vi "Begin.vi"() -> (0 "error out":errorcluster)   [LabVIEW 2013]
doc: "Called before other user functions, this VI is expected to open initial I/O refnums, load in file data, and do all program initialization. Notice that the <B>error out</B> terminal is simply used for data flow. Wiring it to other structures or subVIs ensures that this VI runs first."
uses:
  <vilib>/Rock Robotics/SystemInterfaces/DIO/FPGA_DIOPWMChannel.ctl
  <vilib>/Rock Robotics/WPI/DriverStation/WPI_DriverStationRobotMode2.ctl
  <vilib>/Rock Robotics/WPI/Joystick/WPI_JoystickDeviceEnum.ctl
  <vilib>/Rock Robotics/WPI/SafetyOutput/WPI_SafetyOutputConfigMenu.ctl
  <vilib>/Rock Robotics/SystemInterfaces/DIO/FPGA_DIORelayChannel.ctl
  <vilib>/Rock Robotics/SystemInterfaces/DIO/FPGA_DIOChannel.ctl
  <vilib>/Rock Robotics/SystemInterfaces/Typedef/FPGA_TypedefDigitalModule.ctl
  <vilib>/Rock Robotics/WPI/RobotDrive/WPI_RobotDriveOpen2MotorWithTalon.vi
  Robot Global Data.vi
  <vilib>/Rock Robotics/WPI/Compressor/WPI_CompressorGetSetRefNum.vi
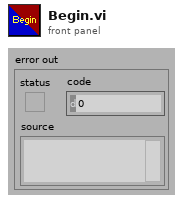
[diagram p1: front panel]
types:
  T1 = typedef "FPGA_TypedefDigitalModule.ctl" = enum16{"Digital Module 1", "Digital Module 2"}
  T2 = typedef "FPGA_DIOChannel.ctl" = enum8{"DIO 1", "DIO 2", "DIO 3", "DIO 4", "DIO 5", "DIO 6", "DIO 7", "DIO 8", "DIO 9", "DIO 10", "DIO 11", "DIO 12", "DIO 13", "DIO 14", "Invalid"}
  T3 = typedef "FPGA_DIORelayChannel.ctl" = enum8{"Relay 1", "Relay 2", "Relay 3", "Relay 4", "Relay 5", "Relay 6", "Relay 7", "Relay 8", "Invalid"}
  T4 = typedef "WPI_SafetyOutputConfigMenu.ctl" = enum16{"Enable", "Disable"}
  T5 = typedef "FPGA_DIOPWMChannel.ctl" = enum8{"PWM 1", "PWM 2", "PWM 3", "PWM 4", "PWM 5", "PWM 6", "PWM 7", "PWM 8", "PWM 9", "PWM 10", "Invalid"}
  T6 = typedef "WPI_JoystickDeviceEnum.ctl" = enum16{"USB 1", "USB 2", "USB 3", "USB 4", "Kinect 1", "Kinect 2"}
  T7 = typedef "WPI_DriverStationRobotMode2.ctl" = enum16{"Autonomous Disabled", "Autonomous Enabled", "Teleop Disabled", "Teleop Enabled", "Timeout", "Finish", "Test Disabled", "Test Enabled"}
  T8 = typedef "WPI_RobotDriveDevRef.ctl" = cluster{"DevStatus":errorcluster, "Motors[]":T9[], "Square Inputs":bool, "Max Output":dbl, "Isochronous":bool}
  T9 = typedef "WPI_MotorControlDeviceRef.ctl" = cluster{"DeviceStatus":errorcluster, "Type":enum16{"PWM", "CAN"}, "PWM":cluster{"Digital Module":T1, "PWM Channel":T5, "DeadBand":T10}, "CAN":cluster{"Device Number":u8, "Control Mode":T11, "Semaphore":T12, "Max Vout":dbl}, "Invert":bool, "TransformRef":T13, "InvTransformRef":T13}
  T10 = typedef "WPI_PWMDeadband.ctl" = cluster{"Name":string, "maxPositivePwm":i32, "minPositivePwm":i32, "centerPwm":i32, "maxNegativePwm":i32, "minNegativePwm":i32, "angularRange":u16}
  T11 = typedef "WPI_CANJaguar_ControlMode.ctl" = enum8{"Percent VBus", "Current", "Speed", "Position", "Voltage"}
  T12 = typedef "Semaphore RefNum" = refnum<k1>
  T13 = typedef "WPI_PWMTransform_ConPane.ctl" = refnum<vi>
  T14 = typedef "WPI_JoystickDevRef.ctl" = cluster{"Device":T6}
  T15 = typedef "WPI_CompressorDevRef.ctl" = cluster{"DevStatus":errorcluster, "DigitalInputDevRef":T16, "RelayDevRef":T17}
  T16 = typedef "WPI_DigitalInputDevRef.ctl" = cluster{"DevStatus":errorcluster, "DIO Channel":T2, "Digital Module":T1}
  T17 = typedef "WPI_RelayDevRef.ctl" = cluster{"DevStatus":errorcluster, "Relay Channel":T3, "Digital Module":T1, "Relay Direction":T18}
  T18 = typedef "WPI_RelayDirection.ctl" = enum16{"Both directions", "Forward only", "Reverse only"}
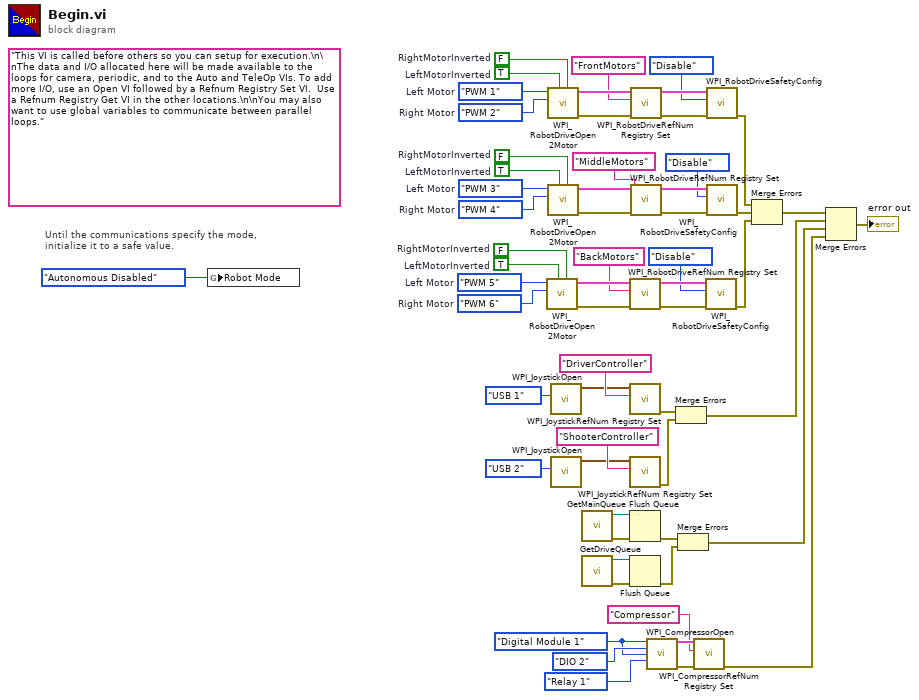
[diagram p0: block diagram]
diagram:
  w1 = FPGA_TypedefDigitalModule."Digital Module 1" ("Pressure Switch\nand Relay Module")
  w26 = FPGA_DIOPWMChannel."PWM 6"  # Right Motor
  w27 = FPGA_DIOPWMChannel."PWM 5"  # Left Motor
  w31 = TRUE  # LeftMotorInverted
  w32 = FALSE  # RightMotorInverted
  w36 = FPGA_DIOPWMChannel."PWM 4"  # Right Motor
  w37 = FPGA_DIOPWMChannel."PWM 3"  # Left Motor
  w41 = TRUE  # LeftMotorInverted
  w42 = FALSE  # RightMotorInverted
  (unwired) "This VI is called before others so you can setup for execution.\n\nThe data and I/O allocated here will be made available to the loops for camera, periodic, and to the Auto and TeleOp VIs. To add more I/O, use an Open VI followed by a Refnum Registry Set VI.  Use a Refnum Registry Get VI in the other locations.\n\nYou may also want to use global variables to communicate between parallel loops."
  w53 = FPGA_DIOPWMChannel."PWM 2"  # Right Motor
  w54 = FPGA_DIOPWMChannel."PWM 1"  # Left Motor
  w58 = TRUE  # LeftMotorInverted
  w59 = FALSE  # RightMotorInverted
  # "Until the communications specify the mode,\ninitialize it to a safe value."
  n1 = global write "Robot Global Data.vi" "Robot Mode"(WPI_DriverStationRobotMode2."Autonomous Disabled" ("Robot Mode")) -> ()
  n2 = call-poly <vilib>:"WPI_RobotDriveOpen2Motor.vi"("Right Motor Inverted"=w32, "Left Motor Inverted"=w31, "Right Motor"=w26, "Left Motor"=w27) -> ("error out"=w28:errorcluster, "RobotDriveDevRef"=w30:T8)  [unwired: 1 in, 5 out]
  n3 = call-poly <vilib>:"WPI_RobotDriveOpen2Motor.vi"("Right Motor Inverted"=w59, "Left Motor Inverted"=w58, "Right Motor"=w53, "Left Motor"=w54) -> ("error out"=w55:errorcluster, "RobotDriveDevRef"=w57:T8)  [unwired: 1 in, 5 out]
  n4 = call-poly <vilib>:"WPI_RobotDriveOpen2Motor.vi"("Right Motor Inverted"=w42, "Left Motor Inverted"=w41, "Right Motor"=w36, "Left Motor"=w37) -> ("error out"=w38:errorcluster, "RobotDriveDevRef"=w40:T8)  [unwired: 1 in, 5 out]
  n5 = call <vilib>:"WPI_JoystickOpen.vi"("JoystickDevice"=WPI_JoystickDeviceEnum."USB 1") -> ("JoystickDevRef"=w48:T14)  [unwired: 10 in]
  n6 = call <vilib>:"WPI_JoystickOpen.vi"("JoystickDevice"=WPI_JoystickDeviceEnum."USB 2") -> ("JoystickDevRef"=w44:T14)  [unwired: 10 in]
  n7 = call "GetMainQueue.vi"() -> ("error out"=w22:errorcluster, "queue out"=w21:refnum<queue>)  [unwired: 10 in]
  n8 = call "GetDriveQueue.vi"() -> ("error out"=w20:errorcluster, "queue out"=w19:refnum<queue>)  [unwired: 10 in]
  n9 = call <vilib>:"WPI_RobotDriveRefNum Registry Set.vi"("error in (no error)"=w28, "refnum name"="BackMotors", "RobotDriveDevRef"=w30) -> ("error out"=w23:errorcluster, "RobotDriveDevRef"=w25:T8)  [unwired: 7 out]
  n10 = call <vilib>:"WPI_JoystickRefNum Registry Set.vi"("refnum name"="DriverController", "JoystickDevRef"=w48) -> ("error out"=w11:errorcluster)  [unwired: 8 in, 1 out]
  n11 = call <vilib>:"WPI_JoystickRefNum Registry Set.vi"("refnum name"="ShooterController", "JoystickDevRef"=w44) -> ("error out"=w10:errorcluster)  [unwired: 8 in, 1 out]
  n12 = Flush Queue(queue=w21, error in (no error)=w22) -> (error out=w9:errorcluster)  [unwired: 2 out]
  n13 = Flush Queue(queue=w19, error in (no error)=w20) -> (error out=w8:errorcluster)  [unwired: 2 out]
  n14 = call <vilib>:"WPI_RobotDriveRefNum Registry Set.vi"("error in (no error)"=w55, "refnum name"="FrontMotors", "RobotDriveDevRef"=w57) -> ("error out"=w46:errorcluster, "RobotDriveDevRef"=w52:T8)  [unwired: 7 out]
  n15 = call <vilib>:"WPI_RobotDriveRefNum Registry Set.vi"("error in (no error)"=w38, "refnum name"="MiddleMotors", "RobotDriveDevRef"=w40) -> ("error out"=w33:errorcluster, "RobotDriveDevRef"=w35:T8)  [unwired: 7 out]
  n16 = call <vilib>:"WPI_CompressorOpen.vi"("Pressure Switch Digital Module (Module 1)"=w1, "Pressure Switch DIO Channel"=FPGA_DIOChannel."DIO 2" ("Pressure Switch Channel"), "Relay Digital Module (Module 1)"=w1, "Relay Channel"=FPGA_DIORelayChannel."Relay 1") -> ("CompressorDevRef"=w17:T15, "error out"=w15:errorcluster)  [unwired: 1 in, 9 out]
  n17 = Merge Errors(w11, w10) -> (w5:errorcluster)
  n18 = Merge Errors(w9, w8) -> (w4:errorcluster)
  n19 = call <vilib>:"WPI_CompressorRefNum Registry Set.vi"("error in (no error)"=w15, "refnum name"="Compressor", "CompressorDevRef"=w17) -> ("error out"=w2:errorcluster)  [unwired: 7 in, 1 out]
  n20 = call <vilib>:"WPI_RobotDriveSafetyConfig.vi"("error in (no error)"=w23, "mode"=WPI_SafetyOutputConfigMenu."Disable", "RobotDriveDevRef"=w25) -> ("error out"=w12:errorcluster)  [unwired: 7 in, 1 out]
  n21 = call <vilib>:"WPI_RobotDriveSafetyConfig.vi"("error in (no error)"=w46, "mode"=WPI_SafetyOutputConfigMenu."Disable", "RobotDriveDevRef"=w52) -> ("error out"=w14:errorcluster)  [unwired: 7 in, 1 out]
  n22 = call <vilib>:"WPI_RobotDriveSafetyConfig.vi"("error in (no error)"=w33, "mode"=WPI_SafetyOutputConfigMenu."Disable", "RobotDriveDevRef"=w35) -> ("error out"=w13:errorcluster)  [unwired: 7 in, 1 out]
  n23 = Merge Errors(w14, w13, w12) -> (w6:errorcluster)
  n24 = Merge Errors(w6, w5, w4, w2) -> (→"error out":errorcluster)
